vi "GeneralGlobals.vi"() -> ()   [LabVIEW 2015]
panel:
  out "DistanceOverride":bool
  out "Ball In Shooter":bool
  out "Reloading":bool
  out "TwoBallAuto":bool
  out "Ball In Roller":bool
  out "ClimberReady":bool
  out "DoneReloading":bool
  out "ShootBall":bool
  out "ManipulatorSelector":i32
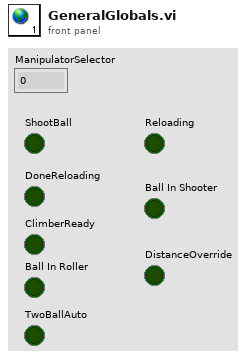
[diagram p1: front panel]
diagram:
